vi "mainVI.vi"() -> ()   [LabVIEW 2019]
uses:
  <vilib>/Platform/TimedLoop/XDataNode/timing_clust.ctl
  <vilib>/Platform/TimedLoop/XDataNode/nitl_modes.ctl
  <vilib>/Platform/TimedLoop/XDataNode/wakeup.ctl
  <extravilib>/ChannelInstances/Tag-bool/Read With Abort.vi
  <extravilib>/ChannelInstances/Tag-bool/Write With Abort.vi
  <vilib>/Plasmionique/MB Master/MB_Master_TCP/MB_Master_TCP.lvclass
  C:/Program Files (x86)/National Instruments/LabVIEW 2019/vi.lib/Plasmionique/MB Master/MB_Master/MB_Master.lvclass
  <extravilib>/ChannelInstances/Tag-bool/Instantiate.vi
  <extravilib>/ChannelInstances/Tag-bool/EndpointRead.vi
  <extravilib>/ChannelInstances/Tag-bool/Endpoint.vi
  <vilib>/Platform/TimedLoop/XDataNode/XDataNode.xnode
  <vilib>/Platform/TimedLoop/XDataNode/XDNodeRunTimeDep.lvlib
  <vilib>/Plasmionique/MB Master/MB Master.lvlib
  <extravilib>/ChannelInstances/Tag-bool.lvlib
panel:
  out "Haute temperature":bool
  in  "Temperature maximale":dbl caption="Fréequence d'échantillonage (Hz)"
  in  "Nom de l'analyse":string="169.254.133.212"
  out "Ready":bool
  in  "START":bool
  in  "stop":bool
  out "Signal de sortie":sgl(graph)
  out "Signal d'entrée mesuré":sgl(graph)
  out "Das trouvé":bool
  out "Signal d'entrée":cluster{dbl[], dbl[]}(graph)
  out "DSP par FFT":cluster{dbl[], dbl[]}(graph)
  out "Alim connectée":bool
  in  "Fréequence \nd'échantillonage (alim)":dbl=1.0 caption="Fréequence d'échantillonage (Hz)"
  in  "Numéro de la machine voulu":string="2196400002"
  in  "Generation de données":enum32{"Labview", "CSV"}(tab)
  in  "Labview opt":T1={"Fréequence maximale (Hz)"=0.1, "Temps de simulation (min)"=2.0, "Amplitude minimale (V)"=0.0, "Amplitude maximale (V)"=1.0}
  in  "Chemin du fichier":path=path "C:/Users/manip/Documents/Thermo aquisition data/labview/input/data.csv"
  out "Machines trouvées":string[][](array[string])=[["COM7", "PSI 9200-25", "2196400002", "06230310", "", "200,0000", "25,0000", "1500,0000", "0,0000", "240,0000", "33", "PSI 9000 Series", "0", "", "", "", "", "V2.31 24.08.2020", "V2.20 20.11.2020", "V1.6.6", "Modbus_RTU"], ["TCPIP0::169.254.133.212::502::SOCKET", "", "", "", "///", "0,000", "0,000", "0,000", "", "", "0", "Ethernet", "0", "", "", "", "", "", "", "", "Can"]]
  out "Sortie d'erreur":errorcluster
  in  "Adresse IP":string="169.254.133.212"
  in  "Fréequence d'échantillonage \n(aquisition)":dbl caption="Fréequence d'échantillonage (Hz)"
  # "Génération des données"
  # "Acquisition des données"
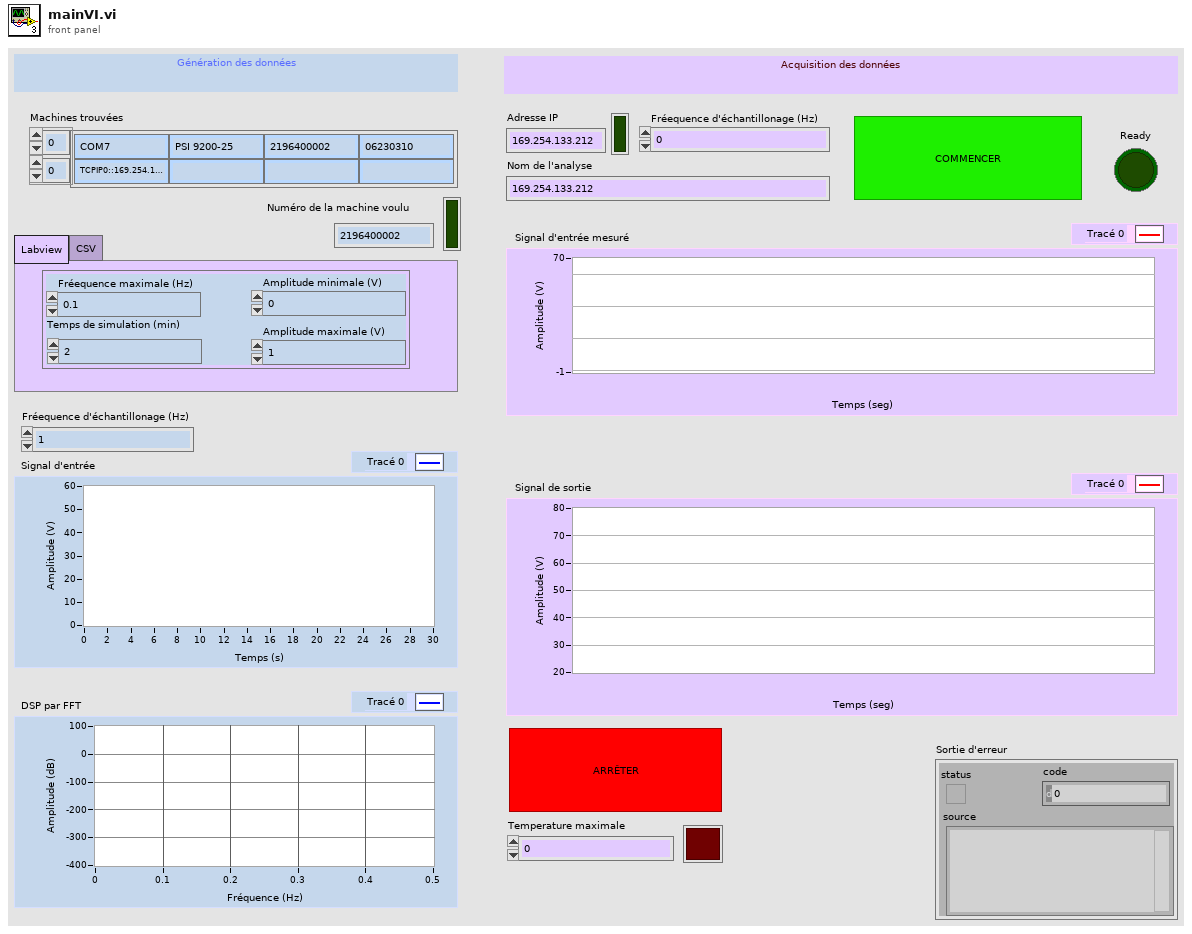
[diagram p1: front panel]
types:
  T1 = cluster{"Fréequence maximale (Hz)":dbl, "Temps de simulation (min)":dbl, "Amplitude minimale (V)":dbl, "Amplitude maximale (V)":dbl}
  T2 = typedef "XDNodeRunTimeDep.lvlib/timing_clust.ctl" = cluster{"Expected End [f-1]":u64, "Actual End [f-1]":u64, "Finished Late? [f-1]":bool, "Expected End [i-1]":u64, "Actual End [i-1]":u64, "Finished Late? [i-1]":bool, "Expected Start [i]":u64, "Actual Start [i]":u64, "Expected Start [f]":u64, "Actual Start [f]":u64, "Source Name":string, "Structure Name":string, "Period":i64, "Deadline":i64, "Offset":i64, "Start":i64, "Priority":i32, "Timeout":i32, "Mode":T3, "Wakeup Reason":T4, "Error":errorcluster, "Source Type":string, "Secondary Source Type":string, "Global End Time":u64, "Global Start Time":u64, "Frame Duration":u64, "Iteration Duration":u64, "Assigned CPU":i32, "I/O Scan Engine Mode":u32}
  T3 = typedef "XDNodeRunTimeDep.lvlib/nitl_modes.ctl" = enum32{"No Change", "Process missed periods, maintain original phase", "Discard missed periods, maintain original phase", "Process missed periods, ignore original phase", "Discard missed periods, ignore original phase"}
  T4 = typedef "XDNodeRunTimeDep.lvlib/wakeup.ctl" = enum32{"Normal", "Aborted", "Asynchronous wakeup", "Timing source error", "Timed loop error", "Timeout"}
  T5 = typedef "Tag-bool.lvlib/))Channel.ctl" = refnum<queue>
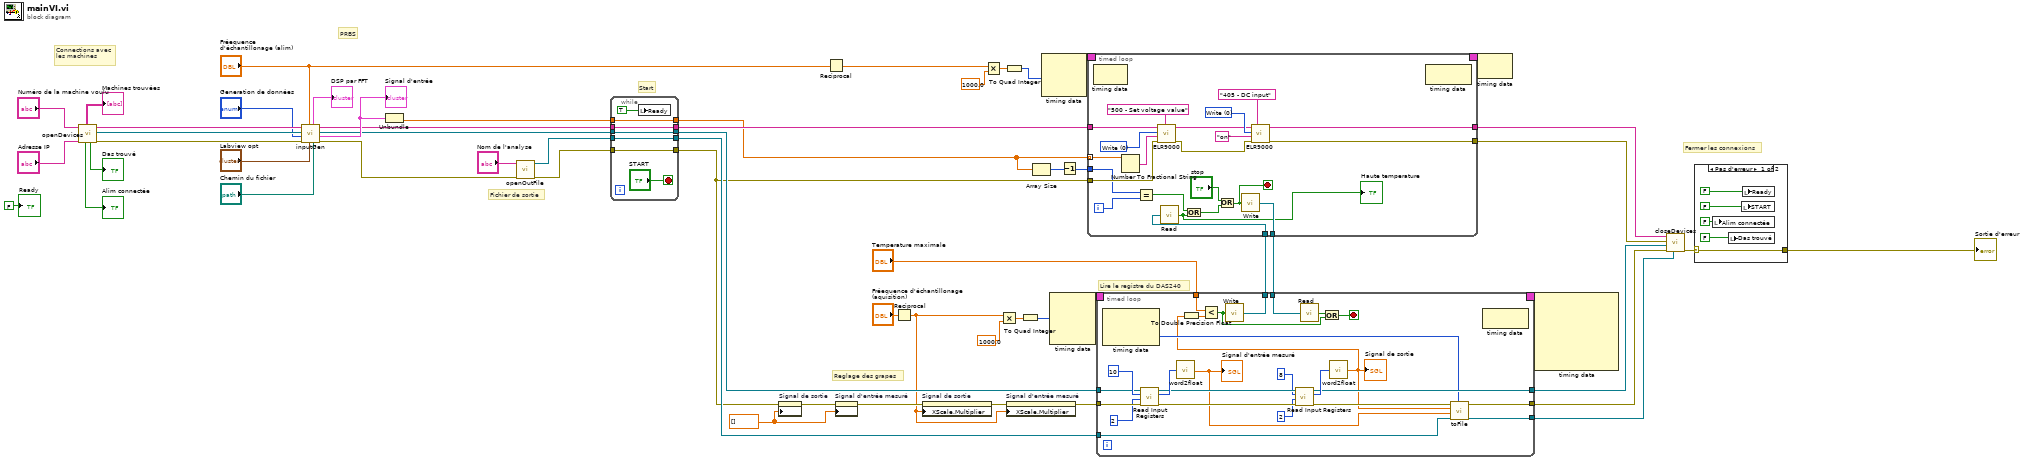
[diagram p0: block diagram]
diagram:
  w6 = sgl[] [] ("Données d'historique")
  # "Reglage des grapes"
  # "Fichier de sortie"
  # "Start"
  # "Fermer les connexions"
  # "Lire le registre du DAS240"
  # "PRBS"
  # "Connections avec\nles machines"
  n1 = call "openDevices.vi"("Adresse IP (DAS240)"="Adresse IP", "Numéro de série (PSI - 9200)"="Numéro de la machine voulu") -> ("Erreur de sortie"=w35:errorcluster, "DAS240_ID"=w37:refnum<class "MB_Master_TCP.lvclass">, "PSI_ID"=w36:string[], "Das trouvé"=→"Das trouvé":bool, "Alim connectée"=→"Alim connectée":bool, "Machines trouvées"=→"Machines trouvées":string[][])  [unwired: 4 in]
  n2 = call "inputGen.vi"("Chemin du fichier"="Chemin du fichier", "Labview opt"="Labview opt", "Fréequence \nd'échantillonage (alim)"="Fréequence \nd'échantillonage (alim)", "Entrée d'erreur"=w35, "Commande onglets"="Generation de données", "DAS240_ID IN"=w37, "PSI_ID IN"=w36) -> ("Sortie d'erreur"=w20:errorcluster, "Signal d'entrée"=w29:cluster{dbl[], dbl[]}, "DAS240_ID OUT"=w24:refnum<class "MB_Master_TCP.lvclass">, "PSI_ID OUT"=w27:string[], "DSP par FFT"=→"DSP par FFT":cluster{dbl[], dbl[]})
  "Signal d'entrée" <- w29
  n3 = Unbundle(w29) -> (w23:dbl[])  [unwired: 1 out]
  n4 = call "openOutFile.vi"("Entrée d'erreur"=w20, "Nom de l'analyse"="Nom de l'analyse") -> ("Sortie d'erreur"=w18:errorcluster, "refnum en sortie"=w16:refnum<file>)  [unwired: 7 in, 1 out]
  n5 = while {
    tunnel: w27 -> [w64]
    tunnel: [w64] -> w26
    tunnel: [w63] -> w25
    tunnel: w24 -> [w63]
    tunnel: [w61] -> w14
    tunnel: w23 -> [w61]
    tunnel: [w60] -> w8
    tunnel: w18 -> [w60]
    tunnel: [w58] -> w17
    tunnel: w16 -> [w58]
    stop <- "START" stop-if-true
    n6 = local write "Ready"(TRUE ("START")) -> ()
  }
  n7 = property on="Signal de sortie" class="GraphDér (strict)"(error in=w8, "History Data"=w6) -> (error out=w7:errorcluster)  [unwired: 1 in, 1 out]
  n8 = Reciprocal(x="Fréequence \nd'échantillonage (alim)") -> (1/x=w4:dbl)
  n9 = property on="Signal d'entrée mesuré" class="GraphDér (strict)"(error in=w7, "History Data"=w6) -> (error out=w5:errorcluster)  [unwired: 1 in, 1 out]
  n10 = Reciprocal(x="Fréequence d'échantillonage \n(aquisition)") -> (1/x=w1:dbl)
  n11 = property on="Signal de sortie" class="GraphDér (strict)"(error in=w5, "XScale.Multiplier"=w1) -> (error out=w2:errorcluster)  [unwired: 1 in, 1 out]
  n12 = Multiply(x=w4, y=1000.0) -> (x*y=w54:dbl)
  n13 = Multiply(x=w1, y=1000.0) -> (x*y=w49:dbl)
  n14 = To Quad Integer(1:w54) -> (0:w53:i64)
  n15 = property on="Signal d'entrée mesuré" class="GraphDér (strict)"(error in=w2, "XScale.Multiplier"=w1) -> (error out=w3:errorcluster)  [unwired: 1 in, 1 out]
  n16 = To Quad Integer(1:w49) -> (0:w47:i64)
  n17 = Array Size(array=w14) -> (size(s)=w13:i32)
  n18 = node-c288(w53) -> (w57:T2)  [unwired: 2 in]
  n19 = node-c288(w47) -> (w52:T2)  [unwired: 3 in]
  n20 = Decrement(x=w13) -> (x-1=w12:i32)
  n21 = timed-loop {
    timing: w57 -> [_]
    timing-out: [_] -> w56
    tunnel: w26 -> [w76]
    tunnel: w8 -> [w78]
    tunnel: [w66] -> w40
    tunnel: [w77] -> w41
    tunnel: w14 -> [w75] mode=indexing
    tunnel: [w74] -> w28
    tunnel: w12 -> [w73]
    tunnel: w11 -> [w67]
    i -> [w72]
    stop <- w71 stop-if-true
    w84 = u8 0 items=["Write", "Read"] ("Access")
    w86 = u8 0 items=["Write", "Read"] ("Access")
    n22 = node-c288() -> ()  [unwired: 1 in, 1 out]
    n23 = Number To Fractional String(number=w75) -> (F-format string=w79:string)  [unwired: 3 in]
    n24 = Equal?(x=w73, y=w72) -> (x = y?=w68:bool)
    n25 = call <instrlib>:"ELR9000.vi"("Command list"="500 - Set voltage value", "Error in"=w78, "Value"=w79, "Access"=w86, "Device information in"=w76) -> ("Error out"=w81:errorcluster, "Device information out"=w82:string[])  [unwired: 1 in, 2 out]
    n26 = call <extravilib>:"Read.vi"("channel"=w67) -> ("element"=w65:bool)  [unwired: 1 in, 1 out]
    "Haute temperature" <- w65
    n27 = Or(x=w68, y=w65) -> (x .or. y?=w69:bool)
    n28 = Or(x="stop", y=w69) -> (x .or. y?=w71:bool)
    n29 = call <extravilib>:"Write.vi"("element"=w71) -> ("channel"=w74:T5)  [unwired: 1 out]
    n30 = call <instrlib>:"ELR9000.vi"("Command list"="405 - DC input", "Error in"=w81, "Value"="on", "Access"=w84, "Device information in"=w82) -> ("Error out"=w66:errorcluster, "Device information out"=w77:string[])  [unwired: 1 in, 2 out]
    n31 = node-c288() -> ()  [unwired: 1 in, 1 out]
  }
  n32 = timed-loop {
    timing: w52 -> [_]
    timing-out: [_] -> w51
    tunnel: w25 -> [w105]
    tunnel: w3 -> [w113]
    tunnel: [w101] -> w38
    tunnel: [w107] -> w39
    tunnel: w28 -> [w102]
    tunnel: w17 -> [w99]
    tunnel: [w98] -> w15
    tunnel: [w95] -> w11
    tunnel: "Temperature maximale" -> [w91]
    stop <- w92 stop-if-true
    n33 = node-c288() -> (w96:i64)  [unwired: 1 in, 2 out]
    n34 = call <vilib>:"Read Input Registers.vi"("error in (no error)"=w113, "quantity"=u16 2, "starting address"=u16 10, "MB session in"=w105) -> ("error out"=w108:errorcluster, "Registers"=w109:u16[], "MB session out"=w106:refnum<class "MB_Master_TCP.lvclass">)  [unwired: 5 in]
    n35 = call "word2float.vi"("Tableau d'entrée"=w109) -> ("Float de sortie"=w97:sgl)
    "Signal d'entrée mesuré" <- w97
    n36 = call <vilib>:"Read Input Registers.vi"("error in (no error)"=w108, "quantity"=u16 2, "starting address"=u16 8, "MB session in"=w106) -> ("error out"=w100:errorcluster, "Registers"=w110:u16[], "MB session out"=w107:refnum<class "MB_Master_TCP.lvclass">)  [unwired: 5 in]
    n37 = call <extravilib>:"Read.vi"("channel"=w102) -> ("element"=w94:bool)  [unwired: 1 in, 1 out]
    n38 = call "word2float.vi"("Tableau d'entrée"=w110) -> ("Float de sortie"=w89:sgl)
    "Signal de sortie" <- w89
    n39 = To Double Precision Float(number=w89) -> (double precision float=w90:dbl)
    n40 = Less?(x=w91, y=w90) -> (x < y?=w93:bool)
    n41 = call <extravilib>:"Write.vi"("element"=w93) -> ("channel"=w95:T5)  [unwired: 1 out]
    n42 = Or(x=w94, y=w93) -> (x .or. y?=w92:bool)
    n43 = call "toFile.vi"("Temps t"=w96, "refnum"=w99, "Tension u"=w97, "Temp y"=w89, "entrée d'erreur"=w100) -> ("refnum en sortie"=w98:refnum<file>, "sortie d'erreur"=w101:errorcluster)  [unwired: 5 in]
    n44 = node-c288() -> ()  [unwired: 1 in, 1 out]
  }
  n45 = node-c288(w56) -> ()  [unwired: 1 out]
  n46 = node-c288(w51) -> ()  [unwired: 7 out]
  n47 = call "closeDevices.vi"("Fichier"=w15, "Erreur d'entrée DAS"=w38, "MB TCP session"=w39, "Erreur d'entrée alim"=w40, "Device information in"=w41) -> ("Erreur de sortie"=w22:errorcluster)  [unwired: 6 in]
  n48 = case shown="Pas d'erreur" w22 {
    selector: w22 -> [w121 w122]
    tunnel: [w121 w122] -> w9
    frame No Error {
      n49 = local write "Alim connectée"(FALSE ("element")) -> ()
      n50 = local write "Das trouvé"(FALSE ("element")) -> ()
      n51 = local write "START"(FALSE ("element")) -> ()
      n52 = local write "Ready"(FALSE ("element")) -> ()
    }
    frame Error {
    }
  }
  "Sortie d'erreur" <- w9
  "Ready" <- FALSE ("Ready")
